vi "Init Globals.vi"() -> (0 "error out":errorcluster)   [LabVIEW 2019, in "Useful OAuth VIs.lvlib"]
uses:
  globals.vi
  Useful OAuth VIs/Useful OAuth VIs.lvlib
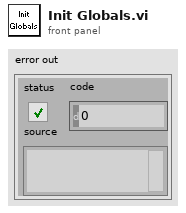
[diagram p1: front panel]
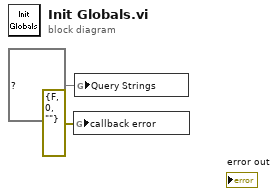
[diagram p0: block diagram]
diagram:
  n1 = global write "globals.vi" "callback error"(errorcluster {"status"=FALSE, "code"=0, "source"=""} ("callback error")) -> ()
  n2 = global write "globals.vi" "Query Strings"(map{string, string} {} ("Query Strings")) -> ()
